vi "CDMA_TxScrambling.vi"(7 "scramble_num_tx":dbl, 8 "error in (no error)":errorcluster caption="错误输入（无错误）", 9 "sc_group_num_tx":dbl, 10 "sf_data":cdb[](array[numeric]), 11 "Path":path) -> (0 "error out":errorcluster caption="错误输出", 2 "sc_data":cdb[](array[numeric]), 3 "Path Out":path)   [LabVIEW 2015]
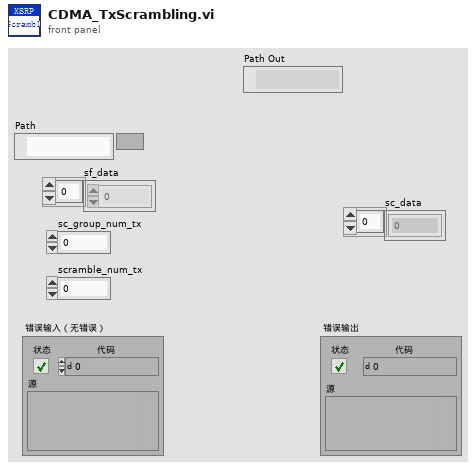
[diagram p1: front panel]
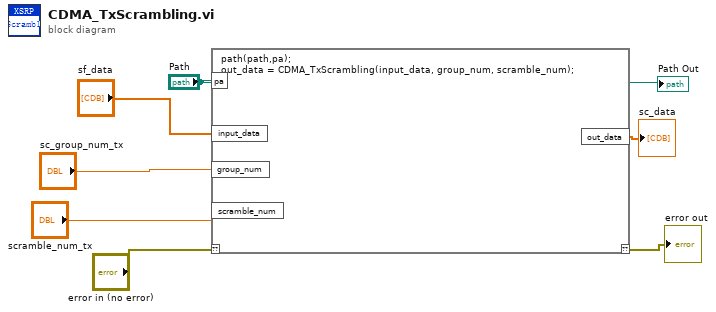
[diagram p0: block diagram]
diagram:
  n1 = script code="path(path,pa);\nout_data = CDMA_TxScrambling(input_data, group_num, scramble_num);"("??"="error in (no error)", "pa"="Path", "input_data"="sf_data", "group_num"="sc_group_num_tx", "scramble_num"="scramble_num_tx") -> ("??"=→"error out":errorcluster, "out_data"=→"sc_data":cdb[])
  "Path Out" <- "Path"
